vi "KGN is connected.vi"(8 "Fehler (Eingang, kein Fehler)":errorcluster, 10 "VISA-Ressourcenname":refnum<visa-resource-name>, 11 "device":u32) -> (0 "Fehler (Ausgang)":errorcluster, 2 "VISA-Ressourcenname out":refnum<visa-resource-name>, 3 "dup device out":u32, 4 "Boolesch":bool)   [LabVIEW 2020, in "Linearisierung v2.lvlib" / "Gasteiler.lvlib" / "HovaCAL_Interface.lvlib" / "KGN.lvlib" / "KGN GUI Get.lvlib"]
uses:
  KGN GUI Get.lvlib
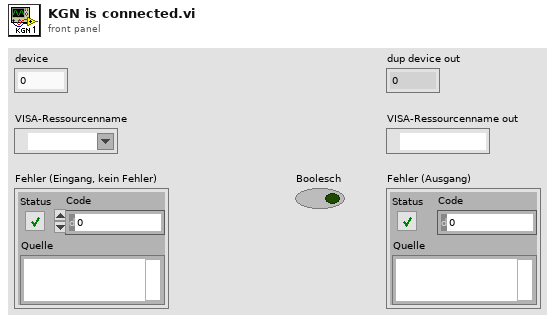
[diagram p1: front panel]
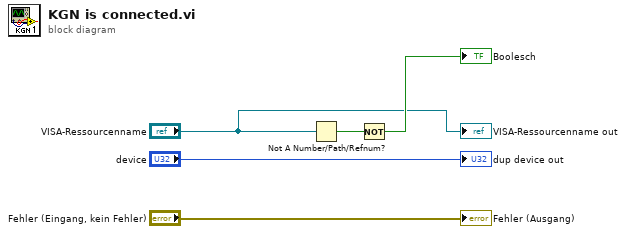
[diagram p0: block diagram]
diagram:
  n1 = Not A Number/Path/Refnum?(number/path/refnum="VISA-Ressourcenname") -> (NaN/Path/Refnum?=w1:bool)
  n2 = Not(x=w1) -> (.not. x?=→"Boolesch":bool)
  "dup device out" <- "device"
  "VISA-Ressourcenname out" <- "VISA-Ressourcenname"
  "Fehler (Ausgang)" <- "Fehler (Eingang, kein Fehler)"
